vi "NodeExist.vi"(8 "error in (no error)":errorcluster caption="错误输入（无错误）", 11 "PanelLinkNode 输入":refnum<class "PanelLinkNode.lvclass"> caption="DNL_LabVIEW Object in") -> (0 "error out":errorcluster caption="错误输出", 1 "Node Exist?":bool, 3 "PanelLinkNode 输出":refnum<class "PanelLinkNode.lvclass"> caption="DNL_LabVIEW Object out")   [LabVIEW 2016, in "PanelLinkNode.lvclass"]
uses:
  PanelLinkNode.lvclass
  PanelObject/PanelObject.lvclass
  PanelLinkNode.lvclass/PanelLinkNode.ctl
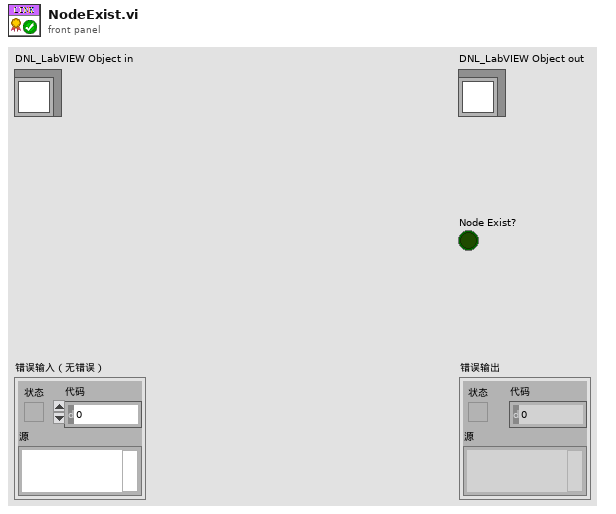
[diagram p1: front panel]
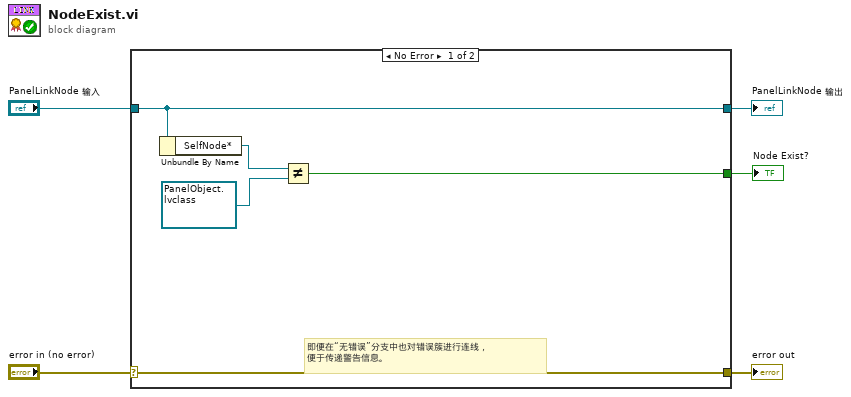
[diagram p0: block diagram]
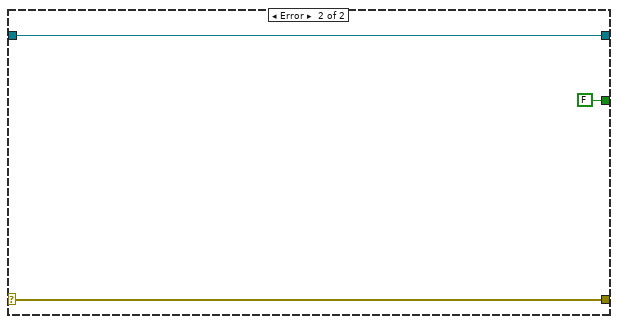
[diagram p2: hidden frame]
diagram:
  n1 = case shown="No Error" "error in (no error)" {
    selector: "error in (no error)" -> [w10 w13]
    tunnel: [w10 w13] -> w4
    tunnel: [w7 w12] -> w2
    tunnel: "PanelLinkNode 输入" -> [w7 w12]
    tunnel: [w8 FALSE] -> w1
    frame No Error {
      # "即便在“无错误”分支中也对错误簇进行连线，\n便于传递警告信息。"
      n2 = Unbundle By Name(w7) -> ("SelfNode*"=w6:refnum<data-value>)
      n3 = Not Equal?(x=w6, y=refnum<data-value> refnum) -> (x != y?=w8:bool)
    }
    frame Error {
    }
  }
  "error out" <- w4
  "PanelLinkNode 输出" <- w2
  "Node Exist?" <- w1
